vi "Handle Events.vi"(8 "error in (no error)":errorcluster, 11 "TreeControlEventHandler":refnum<class "TreeControlEventHandler.lvclass">) -> ()   [LabVIEW 2015, in "ActorEvents.lvlib" / "TreeControlEventHandler.lvclass"]
uses:
  TreeControlEventHandler.lvclass
  IEventHandler/IEventHandler.lvclass/IEventHandler.ctl
  TreeControlEventHandler.lvclass/TreeControlEventHandler.ctl
  <vilib>/ActorFramework/Message Enqueuer/Message Enqueuer.lvclass/Message Enqueuer.ctl
  <vilib>/ActorFramework/Message Priority Queue/Priority Enqueue.vi
  IControlShortcutMenu/IControlShortcutMenu.lvclass
  <vilib>/ActorFramework/Message Enqueuer/Message Enqueuer.lvclass
  IEventAggregator Messages/ValueChangeMsg/ValueChangeMsg.lvclass
  IEventAggregator Messages/ControlMouseDownMsg/ControlMouseDownMsg.lvclass
  IEventAggregator Messages/ControlMouseUpMsg/ControlMouseUpMsg.lvclass
  IEventHandler/IEventHandler.lvclass
  IEventAggregator Messages/TreeItemOpenMsg/TreeItemOpenMsg.lvclass
  IEventAggregator Messages/TreeItemCloseMsg/TreeItemCloseMsg.lvclass
  IEventAggregator Messages/UserShortcutMenuSelectionMsg/UserShortcutMenuSelectionMsg.lvclass
  IEventAggregator Messages/TreeDoubleClickMsg/TreeDoubleClickMsg.lvclass
  IEventAggregator Messages/TreeEditCellMsg/TreeEditCellMsg.lvclass
  IEventAggregator Messages/ShortcutMenuActivationMsg/ShortcutMenuActivationMsg.lvclass
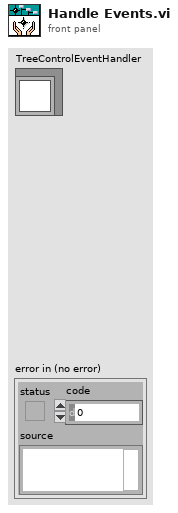
[diagram p1: front panel]
types:
  T1 = typedef "Actor Framework.lvlib/Message Enqueuer.lvclass/Message Priority.ctl" = enum16{"Low", "Normal", "High"}
  T2 = typedef "LVPoint32TypeDef.ctl" = cluster{"Horizontal":i32, "Vertical":i32}
  T3 = cluster{"Shift":bool, "Ctrl":bool, "Alt":bool, "Cmd":bool, "Opt":bool}
  T4 = enum16{"Text", "Background", "Item Symbol", "Open/Close Symbol", "Hierarchy Lines", "Right Border", "Bottom Border", "Bottom Right Corner", "Unknown Part"}
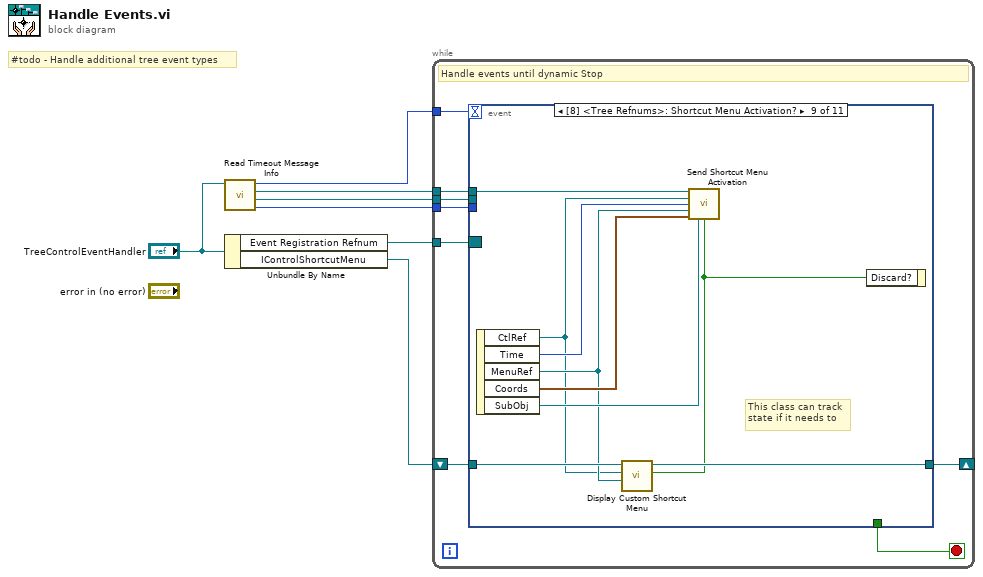
[diagram p0: block diagram]
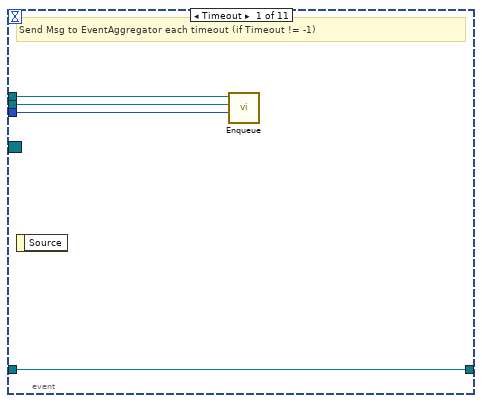
[diagram p2: hidden frame]
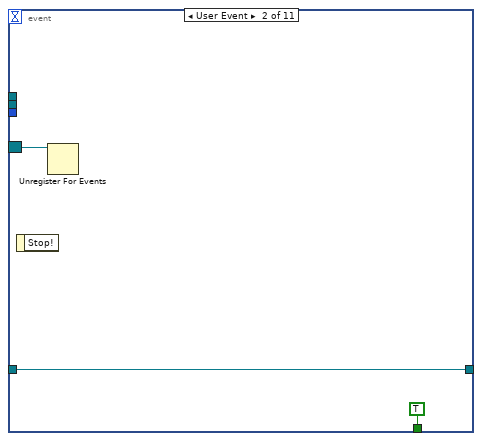
[diagram p3: hidden frame]
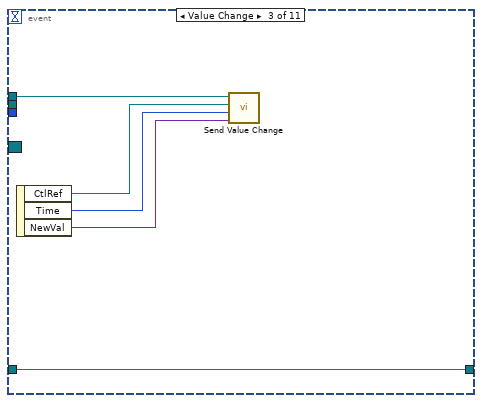
[diagram p4: hidden frame]
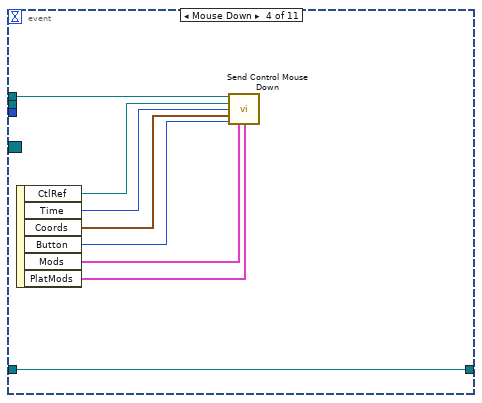
[diagram p5: hidden frame]
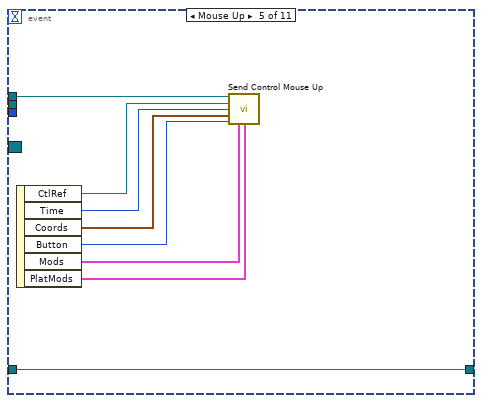
[diagram p6: hidden frame]
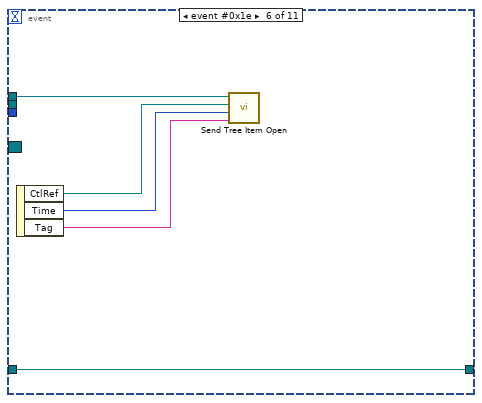
[diagram p7: hidden frame]
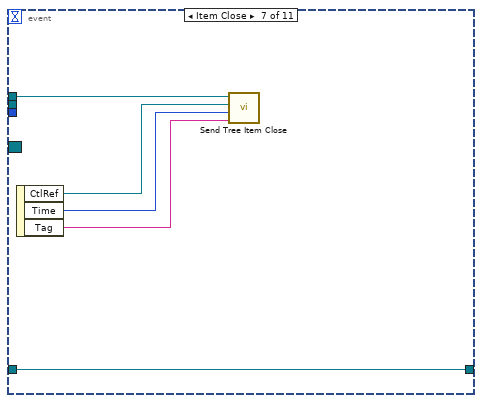
[diagram p8: hidden frame]
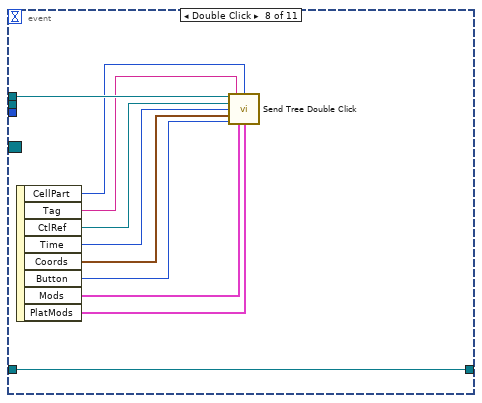
[diagram p9: hidden frame]
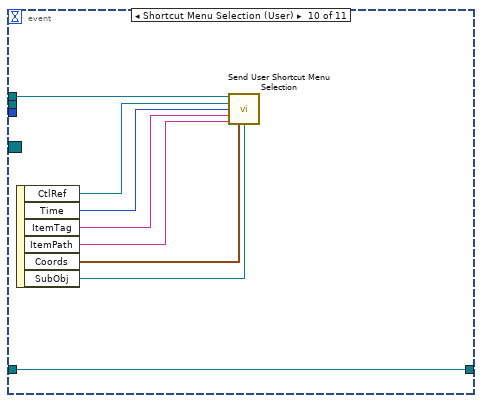
[diagram p10: hidden frame]
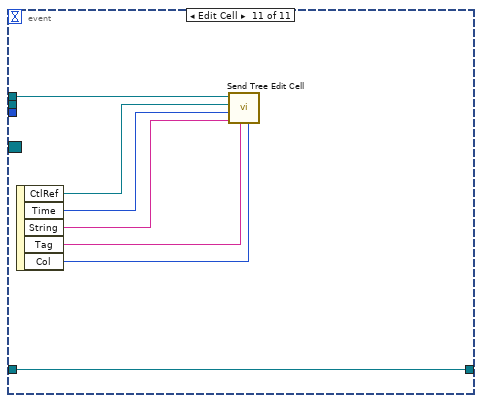
[diagram p11: hidden frame]
diagram:
  # "#todo - Handle additional tree event types"
  n1 = call "Read Timeout Message Info.vi"("IEventHandler in"="TreeControlEventHandler") -> ("Timeout Message Priority"=w4:T1, "Timeout Message"=w5:refnum<class "Message.lvclass">, "EventAggregator Enqueuer"=w6:refnum<class "Message Enqueuer.lvclass">, "Timeout [ms]"=w3:i32)  [unwired: 7 in]
  n2 = Unbundle By Name("TreeControlEventHandler") -> ("Event Registration Refnum"=w7:refnum<event-registration>, "IControlShortcutMenu"=w1:refnum<class "IControlShortcutMenu.lvclass">)
  n3 = while {
    tunnel: w7 -> [w15]
    tunnel: w6 -> [w14]
    tunnel: w5 -> [w13]
    tunnel: w4 -> [w12]
    tunnel: w3 -> [w11]
    shift-right: [w10] -> _
    shift-left: w1 -> [w9]
    stop <- w8 stop-if-true
    # "Handle events until dynamic Stop"
    n4 = event shown="[8] <Tree Refnums>: Shortcut Menu Activation?" {
      selector: w15 -> [_ w22 _ _ _ _ _ _ _ _ _]
      dyn-events: _ -> [_ _ _ _ _ _ _ _ _ _ _]
      timeout: w11 -> [_ _ _ _ _ _ _ _ _ _ _]
      tunnel: [_ TRUE ("Stop!") _ _ _ _ _ _ _ _ _] -> w8
      tunnel: w14 -> [w19 _ w27 w35 w43 w48 w53 w63 w70 w80 w87]
      tunnel: w13 -> [w18 _ _ _ _ _ _ _ _ _ _]
      tunnel: w12 -> [w17 _ _ _ _ _ _ _ _ _ _]
      tunnel: w9 -> [w16 w21 w23 w28 w36 w44 w49 w54 w72 w73 w81]
      tunnel: [w16 w21 w23 w28 w36 w44 w49 w54 w71 w73 w81] -> w10
      event Timeout {
        # "Send Msg to EventAggregator each timeout (if Timeout != -1)"
        n5 = event-data() -> ()  [unwired: 1 in, 1 out]
        n6 = call <vilib>:"Enqueue.vi"("Message Priority (Normal)"=w17, "Message"=w18, "Message Enqueuer in"=w19) -> ()  [unwired: 7 in, 2 out]
      }
      event User Event {
        n7 = event-data() -> ()  [unwired: 1 in, 1 out]
        n8 = Unregister For Events(event registration refnum=w22) -> ()  [unwired: 1 in, 1 out]
      }
      event Value Change {
        n9 = event-data() -> ("CtlRef"=w24:refnum<vi>, "Time"=w26:u32, "NewVal"=w25:variant)  [unwired: 1 in]
        n10 = call "Send Value Change.vi"("New Value"=w25, "Time"=w26, "Ctl Refnum"=w24, "Message Enqueuer in"=w27) -> ()  [unwired: 7 in, 1 out]
      }
      event Mouse Down {
        n11 = event-data() -> ("CtlRef"=w34:refnum<vi>, "Time"=w33:u32, "Coords"=w32:T2, "Button"=w31:u16, "Mods"=w30:cluster{"Double Click":bool, "Menu Key":bool}, "PlatMods"=w29:T3)  [unwired: 1 in]
        n12 = call "Send Control Mouse Down.vi"("Message Enqueuer in"=w35, "Ctl Refnum"=w34, "Time"=w33, "Coords"=w32, "Button"=w31, "Mods"=w30, "PlatMods"=w29) -> ()  [unwired: 8 in, 1 out]
      }
      event Mouse Up {
        n13 = event-data() -> ("CtlRef"=w42:refnum<vi>, "Time"=w41:u32, "Coords"=w40:T2, "Button"=w39:u16, "Mods"=w38:cluster{"Double Click":bool, "Menu Key":bool}, "PlatMods"=w37:T3)  [unwired: 1 in]
        n14 = call "Send Control Mouse Up.vi"("Message Enqueuer in"=w43, "Ctl Refnum"=w42, "Time"=w41, "Coords"=w40, "Button"=w39, "Mods"=w38, "PlatMods"=w37) -> ()  [unwired: 8 in, 1 out]
      }
      event event #0x1e {
        n15 = event-data() -> ("CtlRef"=w47:refnum<vi>, "Time"=w46:u32, "Tag"=w45:string)  [unwired: 1 in]
        n16 = call "Send Tree Item Open.vi"("Item Tag"=w45, "Time"=w46, "Tree Refnum"=w47, "Message Enqueuer in"=w48) -> ()  [unwired: 7 in, 1 out]
      }
      event Item Close {
        n17 = event-data() -> ("CtlRef"=w52:refnum<vi>, "Time"=w51:u32, "Tag"=w50:string)  [unwired: 1 in]
        n18 = call "Send Tree Item Close.vi"("Item Tag"=w50, "Time"=w51, "Tree Refnum"=w52, "Message Enqueuer in"=w53) -> ()  [unwired: 7 in, 1 out]
      }
      event Double Click {
        n19 = event-data() -> ("CellPart"=w55:T4, "Tag"=w56:string, "CtlRef"=w62:refnum<vi>, "Time"=w61:u32, "Coords"=w60:T2, "Button"=w59:u16, "Mods"=w58:cluster{"Double Click":bool, "Menu Key":bool}, "PlatMods"=w57:T3)  [unwired: 1 in]
        n20 = call "Send Tree Double Click.vi"("Message Enqueuer in"=w63, "Tag"=w56, "CellPart"=w55, "Tree Refnum"=w62, "Time"=w61, "Coords"=w60, "Button"=w59, "Mods"=w58, "PlatMods"=w57) -> ()  [unwired: 6 in, 1 out]
      }
      event Shortcut Menu Activation? {
        # "This class can track\nstate if it needs to"
        n21 = event-data() -> ("CtlRef"=w64:refnum<vi>, "Time"=w69:u32, "MenuRef"=w65:refnum<k9>, "Coords"=w68:T2, "SubObj"=w67:refnum<vi>)  [unwired: 1 in]
        n22 = call-dynamic "Display Custom Shortcut Menu.vi"("MenuRef"=w65, "Ctl Refnum"=w64, "IControlShortcutMenu In"=w72) -> ("Discarded?"=w66:bool, "IControlShortcutMenu Out"=w71:refnum<class "IControlShortcutMenu.lvclass">)  [unwired: 6 in, 1 out]
        n23 = call "Send Shortcut Menu Activation.vi"("Message Enqueuer in"=w70, "CtlRef"=w64, "Time"=w69, "MenuRef"=w65, "Coords"=w68, "SubObj"=w67, "Discarded?"=w66) -> ()  [unwired: 8 in, 1 out]
        n24 = event-data("Discard?"=w66) -> ()  [unwired: 1 in, 1 out]
      }
      event Shortcut Menu Selection (User) {
        n25 = event-data() -> ("CtlRef"=w79:refnum<vi>, "Time"=w78:u32, "ItemTag"=w77:string, "ItemPath"=w76:string, "Coords"=w75:T2, "SubObj"=w74:refnum<vi>)  [unwired: 1 in]
        n26 = call "Send User Shortcut Menu Selection.vi"("Message Enqueuer in"=w80, "CtlRef"=w79, "Time"=w78, "Item Tag"=w77, "Item Path"=w76, "Coords"=w75, "SubObj"=w74) -> ()  [unwired: 8 in, 1 out]
      }
      event Edit Cell {
        n27 = event-data() -> ("CtlRef"=w86:refnum<vi>, "Time"=w85:u32, "String"=w84:string, "Tag"=w83:string, "Col"=w82:i32)  [unwired: 1 in]
        n28 = call "Send Tree Edit Cell.vi"("Col"=w82, "Tag"=w83, "String"=w84, "Time"=w85, "CtlRef"=w86, "Message Enqueuer in"=w87) -> ()  [unwired: 5 in, 1 out]
      }
    }
  }
